vi "Auswahlfelder Blinken.vi"(10 "Controls[]":refnum<vi>[](array[refnum])) -> ()   [LabVIEW 2020, in "CalGas Aufschaltung.lvlib"]
uses:
  CalGas Aufschaltung.lvlib
  FGV CalGas Aktionen.ctl
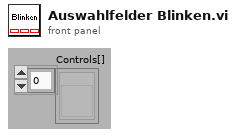
[diagram p1: front panel]
types:
  T1 = typedef "CalGas Aufschaltung.lvlib/FGV CalGas Aktionen.ctl" = enum16{"lesen", "Analysator Auswahl", "Def.CalGas", "Aufschaltung CalGas", "laden", "speichern", "KAL extrahieren"}
  T2 = typedef "CalGas Aufschaltung.lvlib/Aufschaltung CalGas.ctl" = cluster{"Kalibriergas":T3, "Aufschaltpunkt":T4, "Analysator":T5}
  T3 = typedef "Auswahlfeld.ctl" = u16
  T4 = typedef "CalGas Aufschaltung.lvlib/Auswahl Aufschaltpunkt.ctl" = enum16{"über Filterblock", "Analysator direkt", "über PNS", "Entnahme", "Gasdivider"}
  T5 = typedef "CalGas Aufschaltung.lvlib/Auswahl Analysator.ctl" = enum16{"FT-IR", "FID", "PMA", "PMA/FID/FT-IR"}
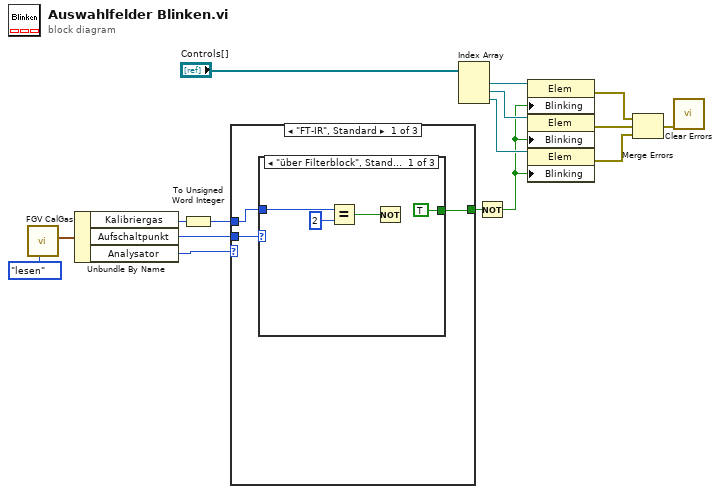
[diagram p0: block diagram]
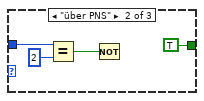
[diagram p2: hidden frame]
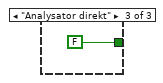
[diagram p3: hidden frame]
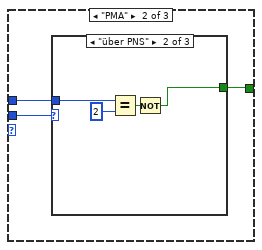
[diagram p4: hidden frame]
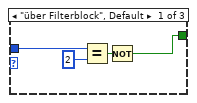
[diagram p5: hidden frame]
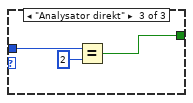
[diagram p6: hidden frame]
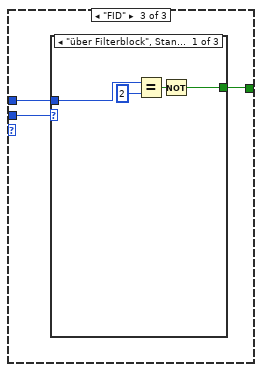
[diagram p7: hidden frame]
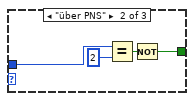
[diagram p8: hidden frame]
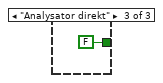
[diagram p9: hidden frame]
diagram:
  n1 = call "FGV CalGas.vi"("Aktionen"=FGV_CalGas_Aktionen."lesen") -> ("Aufschaltung CalGas"=w11:T2)  [unwired: 6 in, 4 out]
  n2 = Unbundle By Name(w11) -> ("Kalibriergas"=w1:T3, "Aufschaltpunkt"=w10:T4, "Analysator"=w9:T5)
  n3 = To Unsigned Word Integer(number=w1) -> (unsigned 16bit integer=w2:T3)
  n4 = case shown="\"FT-IR\", Standard" w9 {
    tunnel: w10 -> [w19 w31 w45]
    tunnel: w2 -> [w17 w30 w44]
    tunnel: [w18 w29 w43] -> w8
    frame "FT-IR", Default {
      n5 = case shown="\"über Filterblock\", Standard" w19 {
        tunnel: [TRUE TRUE FALSE] -> w18
        tunnel: w17 -> [w21 w25 _]
        frame "über Filterblock", Default {
          n6 = Equal?(x=w21, y=u16 2) -> (x = y?=w23:bool)
          n7 = Not(x=w23) -> ()  [unwired: 1 out]
        }
        frame "über PNS" {
          n8 = Equal?(x=w25, y=u16 2) -> (x = y?=w27:bool)
          n9 = Not(x=w27) -> ()  [unwired: 1 out]
        }
        frame "Analysator direkt" {
        }
      }
    }
    frame "PMA" {
      n10 = case shown="\"über PNS\"" w31 {
        tunnel: w30 -> [w34 w36 w40]
        tunnel: [w32 w37 w41] -> w29
        frame "über Filterblock", Default {
          n11 = Equal?(x=w34, y=u16 2) -> (x = y?=w33:bool)
          n12 = Not(x=w33) -> (.not. x?=w32:bool)
        }
        frame "über PNS" {
          n13 = Equal?(x=w36, y=u16 2) -> (x = y?=w38:bool)
          n14 = Not(x=w38) -> (.not. x?=w37:bool)
        }
        frame "Analysator direkt" {
          n15 = Equal?(x=w40, y=u16 2) -> (x = y?=w41:bool)
        }
      }
    }
    frame "FID" {
      n16 = case shown="\"über Filterblock\", Standard" w45 {
        tunnel: w44 -> [w46 w50 _]
        tunnel: [w47 w51 FALSE] -> w43
        frame "über Filterblock", Default {
          n17 = Equal?(x=w46, y=u16 2) -> (x = y?=w49:bool)
          n18 = Not(x=w49) -> (.not. x?=w47:bool)
        }
        frame "über PNS" {
          n19 = Equal?(x=w50, y=u16 2) -> (x = y?=w53:bool)
          n20 = Not(x=w53) -> (.not. x?=w51:bool)
        }
        frame "Analysator direkt" {
        }
      }
    }
  }
  n21 = Index Array(array="Controls[]") -> (element #1=w16:refnum<vi>, element #2=w15:refnum<vi>, element #3=w14:refnum<vi>)  [unwired: 3 in]
  n22 = Not(x=w8) -> (.not. x?=w7:bool)
  n23 = property class="Elem"(reference=w16, "Blinking"=w7) -> (error out=w6:errorcluster)  [unwired: 1 in, 1 out]
  n24 = property class="Elem"(reference=w15, "Blinking"=w7) -> (error out=w5:errorcluster)  [unwired: 1 in, 1 out]
  n25 = property class="Elem"(reference=w14, "Blinking"=w7) -> (error out=w4:errorcluster)  [unwired: 1 in, 1 out]
  n26 = Merge Errors(w6, w5, w4) -> (w3:errorcluster)
  n27 = call <vilib>:"Clear Errors.vi"("error in (no error)"=w3) -> ()  [unwired: 5 in, 2 out]
